vi "MainGUI.vi"(8 "ErrorIn":errorcluster, 11 "OpenCVFaceDetectionIn":refnum<class "OpenCVFaceDetection.lvclass">) -> ()   [LabVIEW 2021, in "OpenCVFaceDetection.lvclass"]
doc: "This is the user interface of the object. It will handle the events to update the GUI."
uses:
  OpenCVFaceDetection.lvclass
  C:/Localdata/Projects/TriekselSoft/TriekselsoftApplicationFramework/Source/.Externals/Library_YAF/YActor/YActor.lvclass
  OpenCVFaceDetection_UiCallBackEvents.ctl
  c1ad68ea-9d58-4aa5-81ea-12a966c9aacc.vi
  OpenCVFaceDetection_ClassCast.vi
  OpenCVFaceDetection.lvclass/OpenCVFaceDetection.ctl
  Library_YAF/YActor/YActor.lvclass
panel:
  out "L_busy":i32
  out "Image":picture
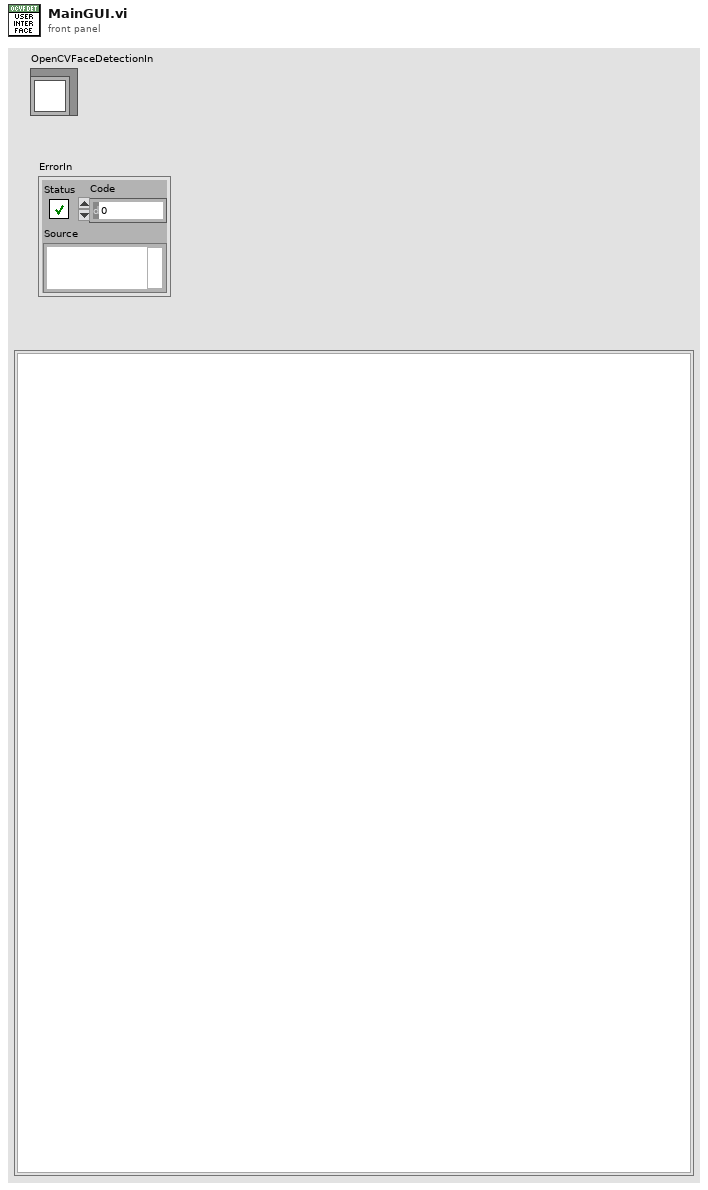
[diagram p1: front panel]
types:
  T1 = typedef "OpenCVFaceDetection.lvclass/OpenCVFaceDetection_UiCallBackEvents.ctl" = enum16{"Default", "PersistentDataUpdated", "NewPicture", "Worker 1: Do Something"}
  T2 = cluster{"Event":string, "This":refnum<class>, "Data":variant}
  T3 = typedef "imagedata.ctl" = cluster{"image type":i32, "image depth":i32, "image":u8[], "mask":u8[], "colors":u32[], "Rectangle":cluster{"left":i16, "top":i16, "right":i16, "bottom":i16}}
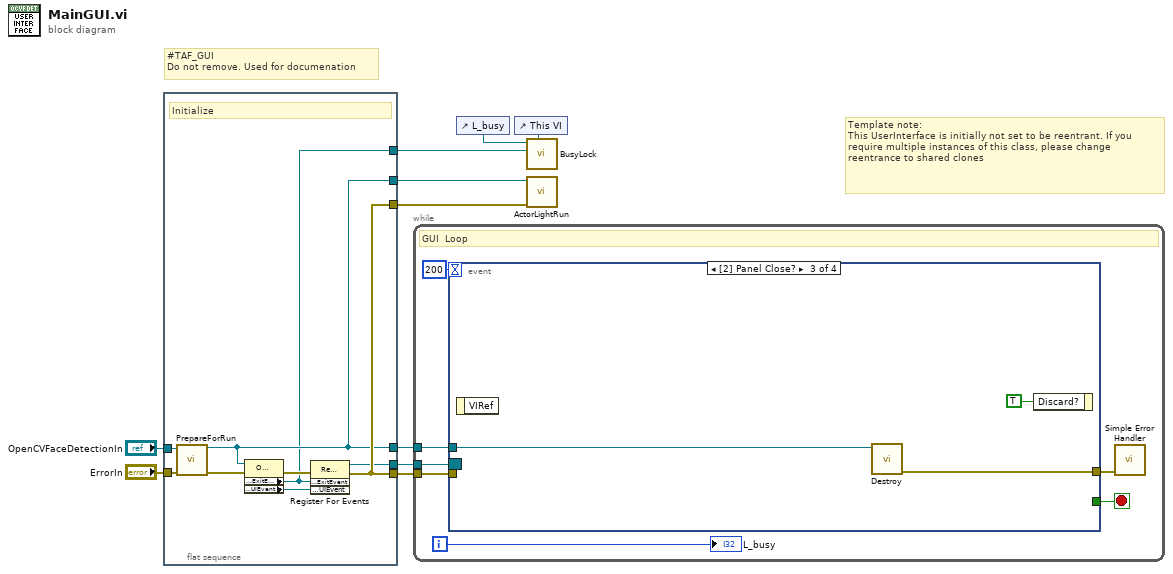
[diagram p0: block diagram]
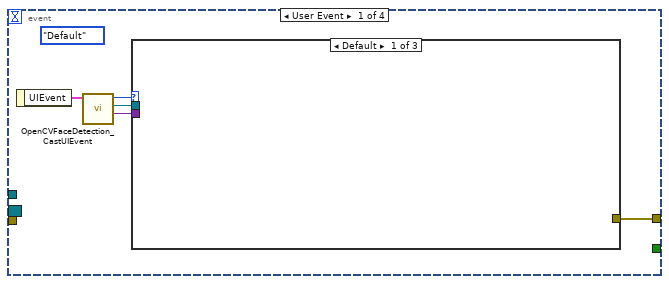
[diagram p2: hidden frame]
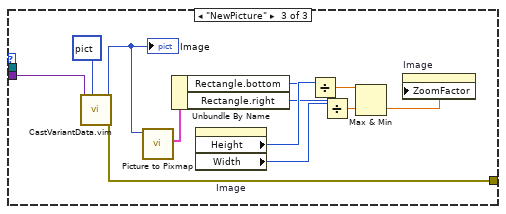
[diagram p4: hidden frame]
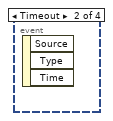
[diagram p5: hidden frame]
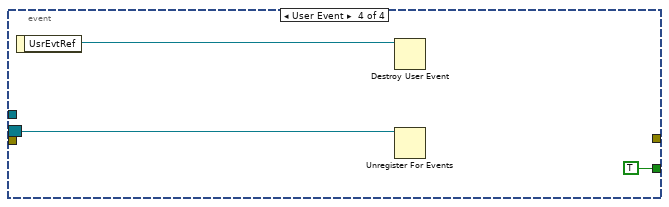
[diagram p6: hidden frame]
diagram:
  # "#TAF_GUI\nDo not remove. Used for documenation"
  # "Template note:\nThis UserInterface is initially not set to be reentrant. If you require multiple instances of this class, please change reentrance to shared clones"
  n1 = flat-sequence {
    tunnel: "ErrorIn" -> [w19]
    tunnel: "OpenCVFaceDetectionIn" -> [w15]
    tunnel: [w14] -> w6
    tunnel: [w11] -> w3
    tunnel: [w13] -> w1
    tunnel: [w16] -> w9
    tunnel: [w13] -> w2
    tunnel: [w16] -> w8
    frame #0 {
      # "Initialize"
      n2 = call-dynamic "PrepareForRun.vi"("ErrorIn"=w19, "YActorIn"=w15) -> ("ErrorOut"=w17:errorcluster, "YActorOut"=w13:refnum<class "OpenCVFaceDetection.lvclass">)  [unwired: 8 in]
      n3 = property class="OpenCVFaceDetection"(reference=w13, error in=w17) -> (error out=w18:errorcluster, "properties:ExitEvent"=w11:refnum<user-event>, "properties:UIEvent"=w12:refnum<user-event>)  [unwired: 1 out]
      n4 = register-events(error in=w18, w11, w12) -> (reference out=w14:refnum<event-registration>, error out=w16:errorcluster)  [unwired: 1 in]
    }
  }
  n5 = while {
    tunnel: w9 -> [w26]
    tunnel: w6 -> [w23]
    tunnel: w1 -> [w20]
    i -> [w22]
    stop <- w24 stop-if-true
    # "GUI  Loop"
    n6 = event shown="[2] Panel Close?" {
      selector: w23 -> [_ _ _ w48]
      dyn-events: _ -> [_ _ _ _]
      timeout: 200 -> [_ _ _ _]
      tunnel: w26 -> [_ _ _ _]
      tunnel: [_ _ _ TRUE] -> w24
      tunnel: [w31 _ w46 _] -> w25
      tunnel: w20 -> [_ _ w44 _]
      event User Event {
        (unwired) OpenCVFaceDetection_UiCallBackEvents."Default" ("UiEventNames")
        n7 = event-data() -> ("UIEvent"=w30:T2)  [unwired: 1 in]
        n8 = call "OpenCVFaceDetection_CastUIEvent.vi"("UIEvent"=w30) -> ("Data"=w27:variant, "ApplicationGUIOut"=w28:refnum<class "OpenCVFaceDetection.lvclass">, "UiEventNames"=w29:T1)  [unwired: 8 in]
        n9 = case shown="Default" w29 {
          tunnel: w28 -> [_ _ _]
          tunnel: w27 -> [_ _ w42]
          tunnel: [_ _ w43] -> w31
          frame Default {
          }
          frame "PersistentDataUpdated" {
            # "Use these events as callbacks from your actor to update the user interface controls. This way your actor will not enter the ui thread, and all UI actions are handled in this VI."
          }
          frame "NewPicture" {
            n10 = call "CastVariantData.vim"("Type"=picture data[5B] ("2D Picture"), "DataIn"=w42) -> ("ErrorOut"=w43:errorcluster, "DataOut"=w33:picture)  [unwired: 8 in]
            "Image" <- w33
            n11 = call <vilib>:"Picture to Pixmap.vi"("picture"=w33) -> ("image data"=w34:T3)  [unwired: 9 in, 1 out]
            n12 = Unbundle By Name(w34) -> ("Rectangle.bottom"=w35:i16, "Rectangle.right"=w36:i16)
            n13 = property on="Image" class="Pict"() -> ("Height"=w39:u32, "Width"=w40:u32)  [unwired: 2 in, 2 out]
            n14 = Divide(x=w39, y=w35) -> (x/y=w38:dbl)
            n15 = Divide(x=w40, y=w36) -> (x/y=w37:dbl)
            n16 = Max & Min(x=w38, y=w37) -> (min(x,y)=w32:dbl)  [unwired: 1 out]
            n17 = property on="Image" class="Pict"("ZoomFactor"=w32) -> ()  [unwired: 2 in, 2 out]
          }
        }
      }
      event Timeout {
        n18 = event-data() -> ()  [unwired: 1 in, 3 out]
      }
      event Panel Close? {
        n19 = event-data() -> ()  [unwired: 1 in, 1 out]
        n20 = call-dynamic "Destroy.vi"("ObjectIn"=w44) -> ("ErrorOut"=w46:errorcluster)  [unwired: 9 in, 1 out]
        n21 = event-data("Discard?"=TRUE) -> ()  [unwired: 1 in, 1 out]
      }
      event User Event {
        n22 = event-data() -> ("UsrEvtRef"=w47:refnum<user-event>)  [unwired: 1 in]
        n23 = Destroy User Event(user event=w47) -> ()  [unwired: 1 in, 1 out]
        n24 = Unregister For Events(event registration refnum=w48) -> ()  [unwired: 1 in, 1 out]
      }
    }
    n25 = call <vilib>:"Simple Error Handler.vi"("error in (no error)"=w25) -> ()  [unwired: 4 in, 5 out]
    "L_busy" <- w22
  }
  n26 = control-ref of="L_busy"() -> (w5:refnum<vi>)
  n27 = control-ref of="This VI"() -> (w4:refnum<vi>)
  n28 = call "BusyLock.vi"("BusyLock"=w4, "ExitEvent"=w3, "Counter"=w5) -> ()  [unwired: 9 in]
  n29 = call "ActorLightRun.vi"("ErrorIn"=w8, "YActorIn"=w2) -> ()  [unwired: 8 in, 2 out]
